vi "Timestamp to Unix epoch time.vi"(1 "Precision (ns)":T1=enum."Nanoseconds", 2 "Timestamp":timestamp format="%<%H:%M:%S%3u\n%Y/%m/%d>T") -> (0 "Unix epoch time":u64)   [LabVIEW 2023]
uses:
  Controls/Precision.ctl
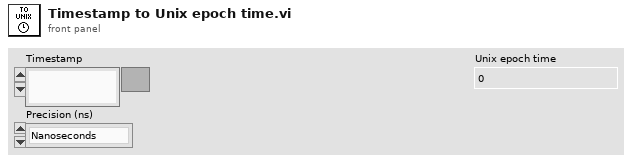
[diagram p1: front panel]
types:
  T1 = typedef "Precision.ctl" = enum16{"Seconds", "Milliseconds", "Nanoseconds"}
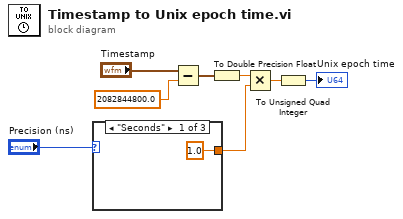
[diagram p0: block diagram]
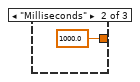
[diagram p2: hidden frame]
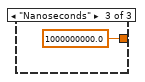
[diagram p3: hidden frame]
diagram:
  n1 = case shown="\"Seconds\"" "Precision (ns)" {
    tunnel: [1.0 ("Database name") 1000.0 ("Database name") 1000000000.0 ("Database name")] -> w2
    frame "Seconds" {
    }
    frame "Milliseconds" {
    }
    frame "Nanoseconds" {
    }
  }
  n2 = Subtract(x="Timestamp", y=2082844800.0) -> (x-y=w5:timestamp)
  n3 = To Double Precision Float(number=w5) -> (double precision float=w7:dbl)
  n4 = Multiply(x=w7, y=w2) -> (x*y=w6:dbl)
  n5 = To Unsigned Quad Integer(1:w6) -> (0:→"Unix epoch time":u64)
